vi "Send Alg Command.vi"(8 "error in":errorcluster, 10 "BusB Serial Port":refnum<visa-resource-name>, 11 "BusB Hardware Configuration.BusB Initialization Parameters":T1) -> (0 "error out":errorcluster, 2 "BusB Serial Port out":refnum<visa-resource-name>, 3 "BusB Hardware Configuration.BusB Initialization Parameters 2":T1)   [LabVIEW 2016, in "Impedance Data Acquisition and Decoding.lvlib"]
uses:
  Impedance Data Acquisition and Decoding.lvlib
  BusB Initialization Parameters.ctl
panel:
  in  "BusB Initialization Parameters":T1
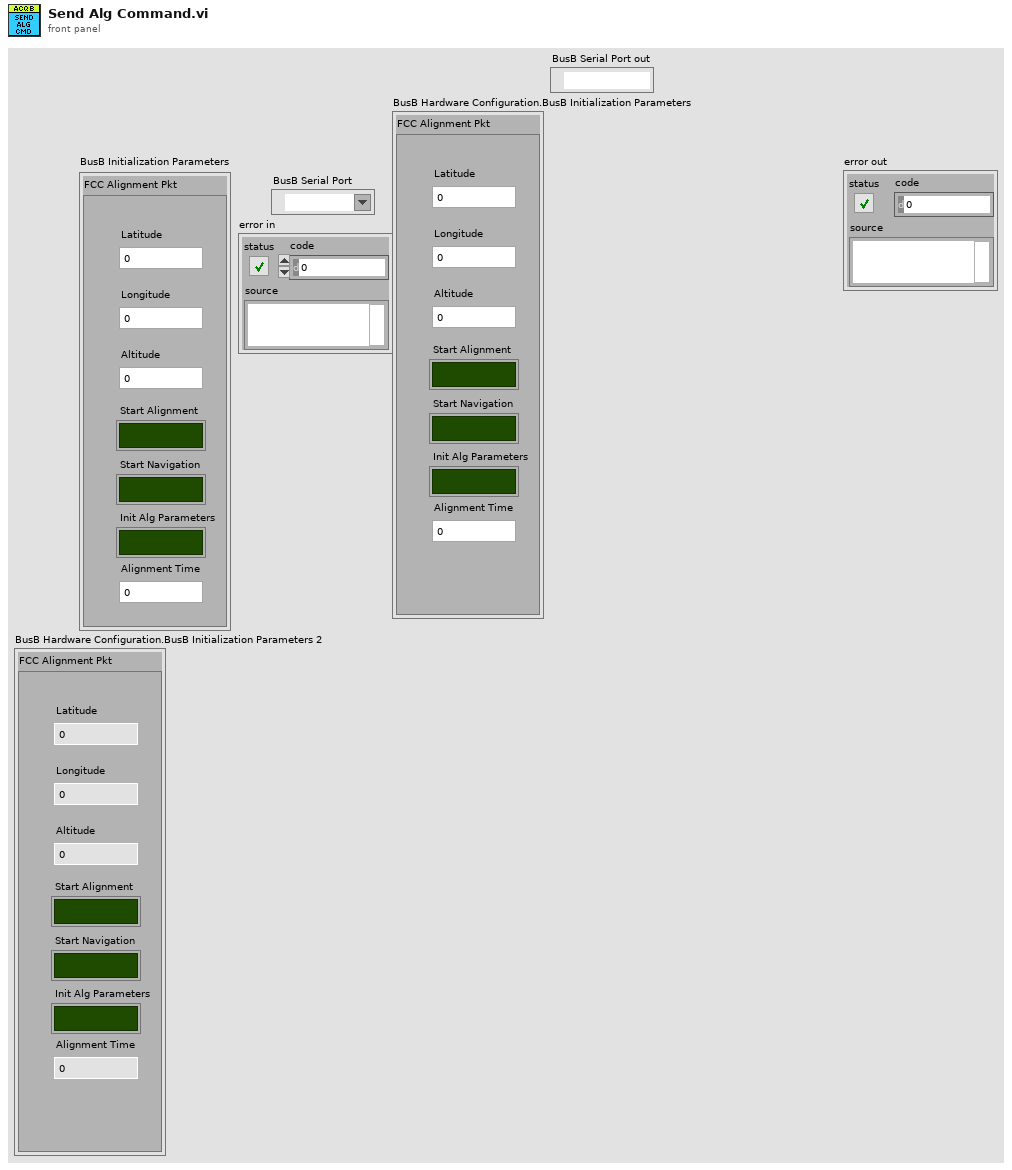
[diagram p1: front panel]
types:
  T1 = typedef "Impedance Data Acquisition and Decoding.lvlib/BusB Initialization Parameters.ctl" = cluster{"FCC Alignment Pkt":cluster{"Latitude":dbl, "Longitude":dbl, "Altitude":dbl, "Start Alignment":bool, "Alignment Time":u8, "Start Navigation":bool, "Init Alg Parameters":bool}}
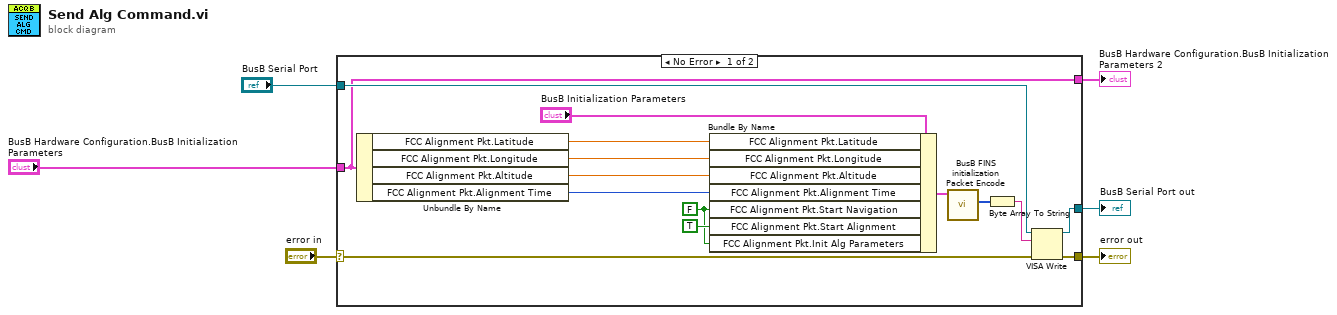
[diagram p0: block diagram]
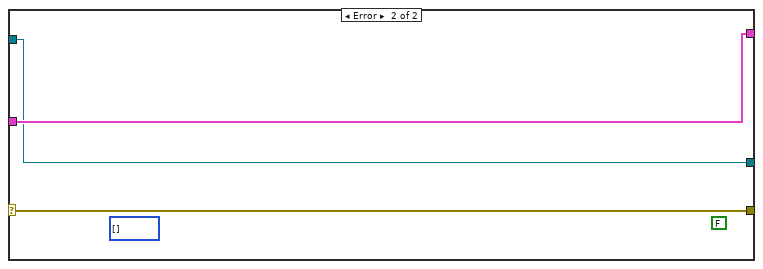
[diagram p2: hidden frame]
diagram:
  n1 = case shown="No Error" "error in" {
    selector: "error in" -> [w21 w24]
    tunnel: [w20 w24] -> w4
    tunnel: "BusB Hardware Configuration.BusB Initialization Parameters" -> [w10 w23]
    tunnel: [w10 w23] -> w1
    tunnel: "BusB Serial Port" -> [w11 w22]
    tunnel: [w9 w22] -> w3
    frame No Error {
      w7 = FALSE
      n2 = Unbundle By Name(w10) -> ("FCC Alignment Pkt.Latitude"=w17:dbl, "FCC Alignment Pkt.Longitude"=w16:dbl, "FCC Alignment Pkt.Altitude"=w15:dbl, "FCC Alignment Pkt.Alignment Time"=w14:u8)
      n3 = Bundle By Name(cluster="BusB Initialization Parameters", "FCC Alignment Pkt.Latitude"=w17, "FCC Alignment Pkt.Longitude"=w16, "FCC Alignment Pkt.Altitude"=w15, "FCC Alignment Pkt.Alignment Time"=w14, "FCC Alignment Pkt.Start Navigation"=w7, "FCC Alignment Pkt.Start Alignment"=TRUE ("FCC Alignment Pkt.Start Navigation"), "FCC Alignment Pkt.Init Alg Parameters"=w7) -> (w13:T1)
      n4 = call "BusB FINS initialization Packet Encode.vi"("BusB Initialization Parameters"=w13) -> ("FCC Navigation send byte Array"=w12:u8[])  [unwired: 8 in, 2 out]
      n5 = Byte Array To String(unsigned byte array=w12) -> (string=w19:string)
      n6 = VISA Write(VISA resource name=w11, write buffer=w19, error in (no error)=w21) -> (VISA resource name out=w9:refnum<visa-resource-name>, error out=w20:errorcluster)  [unwired: 1 out]
    }
    frame Error {
      (unwired) u8[] [] ("Array out")
      (unwired) FALSE
    }
  }
  "error out" <- w4
  "BusB Serial Port out" <- w3
  "BusB Hardware Configuration.BusB Initialization Parameters 2" <- w1
